vi "TDK正向工况电流-继电器控制.vi"() -> ()   [LabVIEW 2021]
uses:
  <vilib>/Utility/file.llb/Read Delimited Spreadsheet (DBL).vi
  <instrlib>/TDK-Lambda G Series/TDK-Lambda G Series.lvlib
panel:
  in  "Voltage Level (0.0 V)":dbl=5.0 format="%#_13g"
  in  "精度":i16
  out "?":bool
  in  "电源台数":dbl=3.0
  in  "TDK地址":refnum<visa-resource-name>="COM15"
  in  "工况2循环次数":i32
  in  "file path (dialog if empty) 2":path caption="工况2"
  out "工况2":string[][](table)
  out "工况1":string[][](table)
  in  "file path (dialog if empty)":path caption="工况1"
  out "已成大循环数":i32
  out "完成工况2循环":i32
  out "完成工况1循环":i32
  in  "工况切换地址":refnum<visa-resource-name>
  in  "停止":bool
  in  "工况1循环次数":i32
  in  "大循环次数":i32
  in  "工况2":cluster{"CH1":bool, "CH2":bool}
  in  "工况1":cluster{"CH1":bool, "CH2":bool}
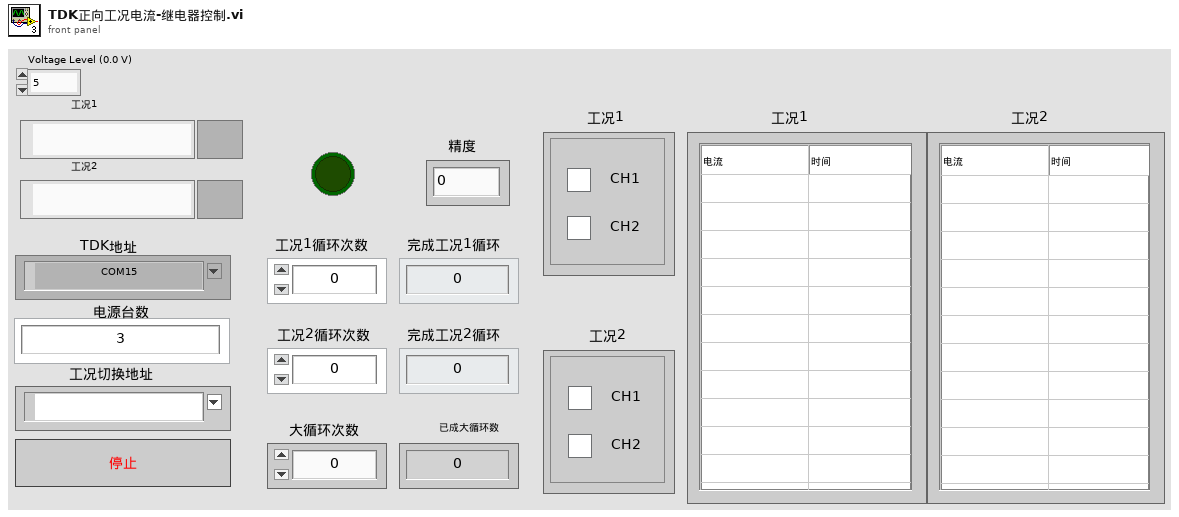
[diagram p1: front panel]
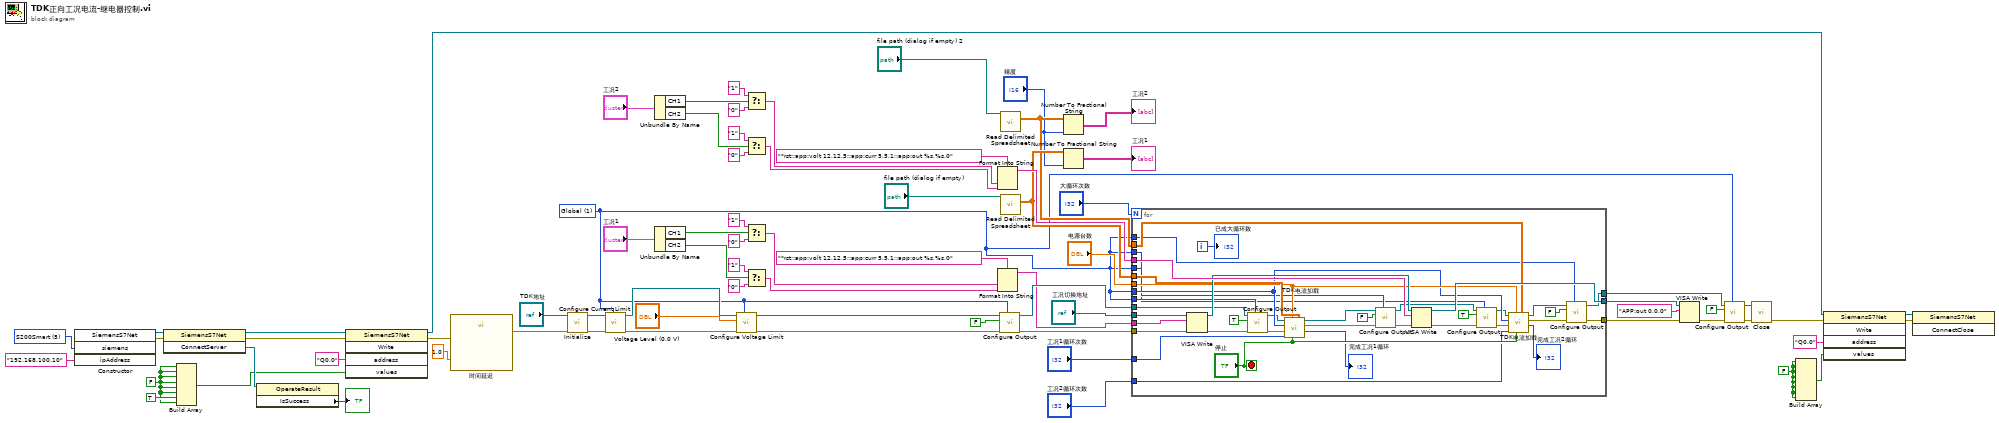
[diagram p0: block diagram]
diagram:
  w8 = FALSE ("元素")
  w17 = FALSE ("元素")
  w19 = 5 items=["S1200"=1, "S300"=2, "S400"=3, "S1500"=4, "S200Smart"=5, "S200"=6] ("siemens")
  w4 = u16 1 items=["Single", "Global"] ("Globalize (0: Single)")
  n1 = constructor class="SiemensS7Net"("siemens"=w19, "ipAddress"="192.168.100.10") -> (reference out=w26:refnum<k24>, error out=w27:errorcluster)  [unwired: 3 in, 3 out]
  n2 = invoke class="SiemensS7Net" method="ConnectServer"(reference=w26, error in=w27) -> (reference out=w22:refnum<k24>, error out=w21:errorcluster, "ConnectServer"=w24:refnum<k24>)  [unwired: 1 in]
  n3 = Build Array(w17, w17, w17, w17, w17, w17, TRUE ("元素"), w17) -> (w20:bool[])
  n4 = property class="OperateResult"(reference=w24) -> ("IsSuccess"=→"?":bool)  [unwired: 1 in, 2 out]
  n5 = invoke class="SiemensS7Net" method="Write"(reference=w22, error in=w21, "address"="Q0.0", "values"=w20) -> (reference out=w12:refnum<k24>, error out=w2:errorcluster)  [unwired: 1 in, 3 out]
  n6 = call "时间延迟"("error in (no error)"=w2, "Delay Time (s)"=1.0) -> ("error out"=w1:errorcluster)  [unwired: 9 in]
  n7 = call <instrlib>:"Initialize.vi"("error in (no error)"=w1, "VISA resource name"="TDK地址") -> ("error out"=w40:errorcluster, "VISA resource name out"=w41:refnum<visa-resource-name>)  [unwired: 8 in]
  n8 = call <instrlib>:"Configure Current Limit.vi"("Globalize (0: Single)"=w4, "error in (no error)"=w40, "VISA resource name"=w41) -> ("error out"=w39:errorcluster, "VISA resource name out"=w38:refnum<visa-resource-name>)  [unwired: 7 in]
  n9 = Unbundle By Name("工况2") -> ("CH1"=w66:bool, "CH2"=w44:bool)
  n10 = Unbundle By Name("工况1") -> ("CH1"=w75:bool, "CH2"=w45:bool)
  n11 = call <instrlib>:"Configure Voltage Limit.vi"("Globalize (0: Single)"=w4, "error in (no error)"=w39, "Voltage Limit (0V)"="Voltage Level (0.0 V)", "VISA resource name"=w38) -> ("error out"=w36:errorcluster, "VISA resource name out"=w37:refnum<visa-resource-name>)  [unwired: 6 in]
  n12 = Select(t="1", s=w66, f="0") -> (s? t:f=w65:string)
  n13 = Select(t="1", s=w44, f="0") -> (s? t:f=w64:string)
  n14 = Select(t="1", s=w75, f="0") -> (s? t:f=w74:string)
  n15 = Select(t="1", s=w45, f="0") -> (s? t:f=w73:string)
  n16 = Format Into String(format string="*rst;:app:volt 12,12,5;:app:curr 5,5,1;:app:out %s,%s,0" ("格式字符串"), w65, w64) -> (resulting string=w58:string)  [unwired: 2 in, 1 out]
  n17 = Format Into String(format string="*rst;:app:volt 12,12,5;:app:curr 5,5,1;:app:out %s,%s,0" ("格式字符串"), w74, w73) -> (resulting string=w5:string)  [unwired: 2 in, 1 out]
  n18 = call <instrlib>:"Configure Output.vi"("Globalize (0: Single)"=w4, "error in (no error)"=w36, "Enable Output (False)"=FALSE, "VISA resource name"=w37) -> ("error out"=w34:errorcluster, "VISA resource name out"=w33:refnum<visa-resource-name>)  [unwired: 6 in]
  n19 = call-poly <vilib>:"Read Delimited Spreadsheet.vi"("file path (dialog if empty)"="file path (dialog if empty) 2") -> ("all rows"=w49:dbl[][])  [unwired: 9 in, 5 out]
  n20 = call-poly <vilib>:"Read Delimited Spreadsheet.vi"("file path (dialog if empty)"="file path (dialog if empty)") -> ("all rows"=w51:dbl[][])  [unwired: 9 in, 5 out]
  n21 = Number To Fractional String(number=w49, precision (6)="精度") -> (F-format string=→"工况2":string[][])  [unwired: 2 in]
  n22 = Number To Fractional String(number=w51, precision (6)="精度") -> (F-format string=→"工况1":string[][])  [unwired: 2 in]
  n23 = for {
    N: "大循环次数" -> [_]
    tunnel: w5 -> [w115]
    tunnel: "工况切换地址" -> [w114]
    tunnel: w58 -> [w113]
    tunnel: [w111] -> w57
    tunnel: w33 -> [w95]
    tunnel: w51 -> [w110]
    tunnel: w49 -> [w109]
    tunnel: w34 -> [w108]
    tunnel: [w89] -> w15
    tunnel: "工况1循环次数" -> [w103]
    tunnel: "工况2循环次数" -> [w102]
    tunnel: [w87] -> w16
    tunnel: w4 -> [w100]
    tunnel: "电源台数" -> [w101]
    tunnel: w4 -> [w84]
    tunnel: w4 -> [w83]
    tunnel: w4 -> [w82]
    tunnel: w4 -> [w81]
    i -> [w104]
    stop <- "停止" stop-if-true
    n24 = VISA Write(VISA resource name=w114, write buffer=w115, error in (no error)=w108) -> (VISA resource name out=w112:refnum<visa-resource-name>, error out=w99:errorcluster)  [unwired: 1 out]
    n25 = call <instrlib>:"Configure Output.vi"("Globalize (0: Single)"=w84, "error in (no error)"=w99, "Enable Output (False)"=TRUE, "VISA resource name"=w95) -> ("error out"=w98:errorcluster, "VISA resource name out"=w88:refnum<visa-resource-name>)  [unwired: 6 in]
    n26 = call "TDK电流加载.vi"("all rows"=w110, "停止"="停止", "电源台数"=w101, "循环次数"=w103, "error out"=w98, "Globalize (0: Single)"=w100, "VISA resource name out"=w88) -> ("已完成循环次数"=→"完成工况1循环":i32, "error out 2"=w80:errorcluster, "VISA resource name out 2"=w79:refnum<visa-resource-name>)  [unwired: 2 in]
    n27 = call <instrlib>:"Configure Output.vi"("Globalize (0: Single)"=w83, "error in (no error)"=w80, "Enable Output (False)"=FALSE, "VISA resource name"=w79) -> ("error out"=w96:errorcluster, "VISA resource name out"=w86:refnum<visa-resource-name>)  [unwired: 6 in]
    n28 = VISA Write(VISA resource name=w112, write buffer=w113, error in (no error)=w96) -> (VISA resource name out=w111:refnum<visa-resource-name>, error out=w93:errorcluster)  [unwired: 1 out]
    n29 = call <instrlib>:"Configure Output.vi"("Globalize (0: Single)"=w82, "error in (no error)"=w93, "Enable Output (False)"=TRUE, "VISA resource name"=w86) -> ("error out"=w92:errorcluster, "VISA resource name out"=w85:refnum<visa-resource-name>)  [unwired: 6 in]
    n30 = call "TDK电流加载.vi"("all rows"=w109, "停止"="停止", "电源台数"=w101, "循环次数"=w102, "error out"=w92, "Globalize (0: Single)"=w100, "VISA resource name out"=w85) -> ("已完成循环次数"=→"完成工况2循环":i32, "error out 2"=w78:errorcluster, "VISA resource name out 2"=w77:refnum<visa-resource-name>)  [unwired: 2 in]
    n31 = call <instrlib>:"Configure Output.vi"("Globalize (0: Single)"=w81, "error in (no error)"=w78, "Enable Output (False)"=FALSE, "VISA resource name"=w77) -> ("error out"=w89:errorcluster, "VISA resource name out"=w87:refnum<visa-resource-name>)  [unwired: 6 in]
    "已成大循环数" <- w104
  }
  n32 = VISA Write(VISA resource name=w57, write buffer="APP:out 0,0,0" ("写入缓冲区"), error in (no error)=w15) -> (error out=w28:errorcluster)  [unwired: 2 out]
  n33 = call <instrlib>:"Configure Output.vi"("Globalize (0: Single)"=w4, "error in (no error)"=w28, "Enable Output (False)"=FALSE, "VISA resource name"=w16) -> ("error out"=w30:errorcluster, "VISA resource name out"=w31:refnum<visa-resource-name>)  [unwired: 6 in]
  n34 = call <instrlib>:"Close.vi"("error in (no error)"=w30, "VISA resource name"=w31) -> ("error out"=w10:errorcluster)  [unwired: 9 in]
  n35 = Build Array(w8, w8, w8, w8, w8, w8, w8, w8) -> (w13:bool[])
  n36 = invoke class="SiemensS7Net" method="Write"(reference=w12, error in=w10, "address"="Q0.0", "values"=w13) -> (reference out=w11:refnum<k24>, error out=w9:errorcluster)  [unwired: 1 in, 3 out]
  n37 = invoke class="SiemensS7Net" method="ConnectClose"(reference=w11, error in=w9) -> ()  [unwired: 1 in, 3 out]
